vi "ToString.vi"(8 "error in (no error)":errorcluster, 11 "IsEqual in":refnum<class "IsEqual.lvclass">) -> (0 "error out":errorcluster, 2 "String":string, 3 "IsEqual out":refnum<class "IsEqual.lvclass">)   [LabVIEW 2017, in "Transparent Assertions.lvlib" / "IsEqual.lvclass"]
doc: "Returns a string representation of the object."
uses:
  IsEqual.lvclass
  IsEqual.lvclass/IsEqual.ctl
  To JSON.vi/c34f3794-71bb-4fc1-98c1-2c7c55f09150.vi
  <vilib>/PNR/JSONtext Object Serialization/Generic Object Serializer/Generic Object Serializer.lvclass
  C:/Program Files/National Instruments/LabVIEW 2017/vi.lib/JDP Science/JSONtext/LVClass Serializer/JSONtext LVClass Serializer.lvclass
  <vilib>/JDP Science/JSONtext/Variant to JSON Text.vi
  Transparent Assertions.lvlib
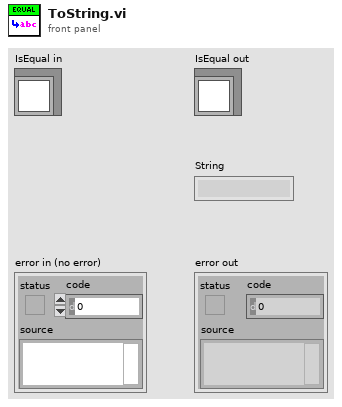
[diagram p1: front panel]
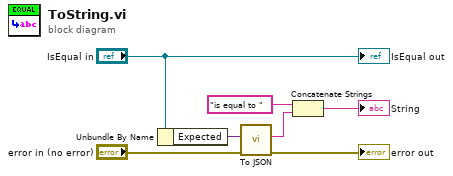
[diagram p0: block diagram]
diagram:
  n1 = Unbundle By Name("IsEqual in") -> ("Expected"=w4:variant)
  n2 = call "To JSON.vi"("error in (no error)"="error in (no error)", "Anything"=w4) -> ("error out"=→"error out":errorcluster, "JSON"=w3:string)  [unwired: 8 in]
  n3 = Concatenate Strings("is equal to " ("String"), w3) -> (→"String":string)
  "IsEqual out" <- "IsEqual in"
